vi "Decode DRV stand (SubVI).vi"(8 "error in (no error)":errorcluster, 9 "Excel Data":string[][](array[string]), 11 "SAP ID":string) -> (0 "error out":errorcluster, 1 "subarray":string[](array[string]), 3 "DRV stand":T1)   [LabVIEW 2018, in "Application.lvlib"]
uses:
  Application/Application.lvlib
  Application/DRV stand.ctl
panel:
  out "DriverID":string
  out "Name":string
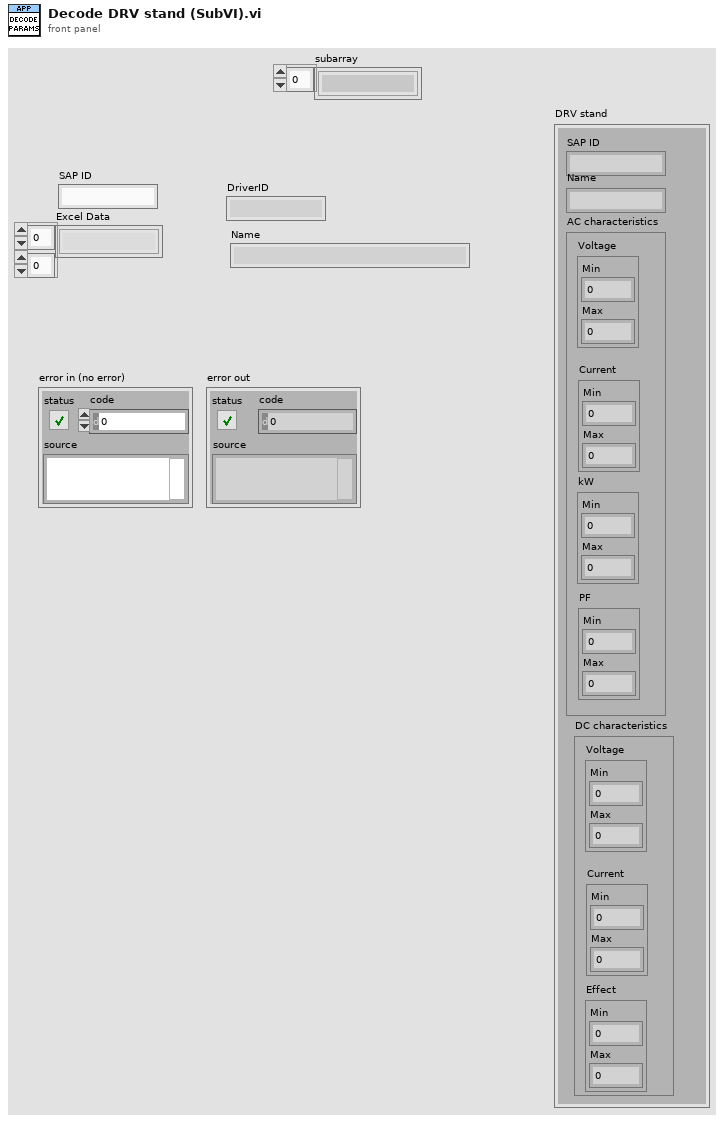
[diagram p1: front panel]
types:
  T1 = typedef "Application.lvlib/DRV stand.ctl" = cluster{"SAP ID":string, "Name":string, "AC characteristics":cluster{"Voltage":cluster{"Min":dbl, "Max":dbl}, "Current":cluster{"Min":dbl, "Max":dbl}, "kW":cluster{"Min":dbl, "Max":dbl}, "PF":cluster{"Min":dbl, "Max":dbl}}, "DC characteristics":cluster{"Voltage":cluster{"Min":dbl, "Max":dbl}, "Current":cluster{"Min":dbl, "Max":dbl}, "Effect":cluster{"Min":dbl, "Max":dbl}}}
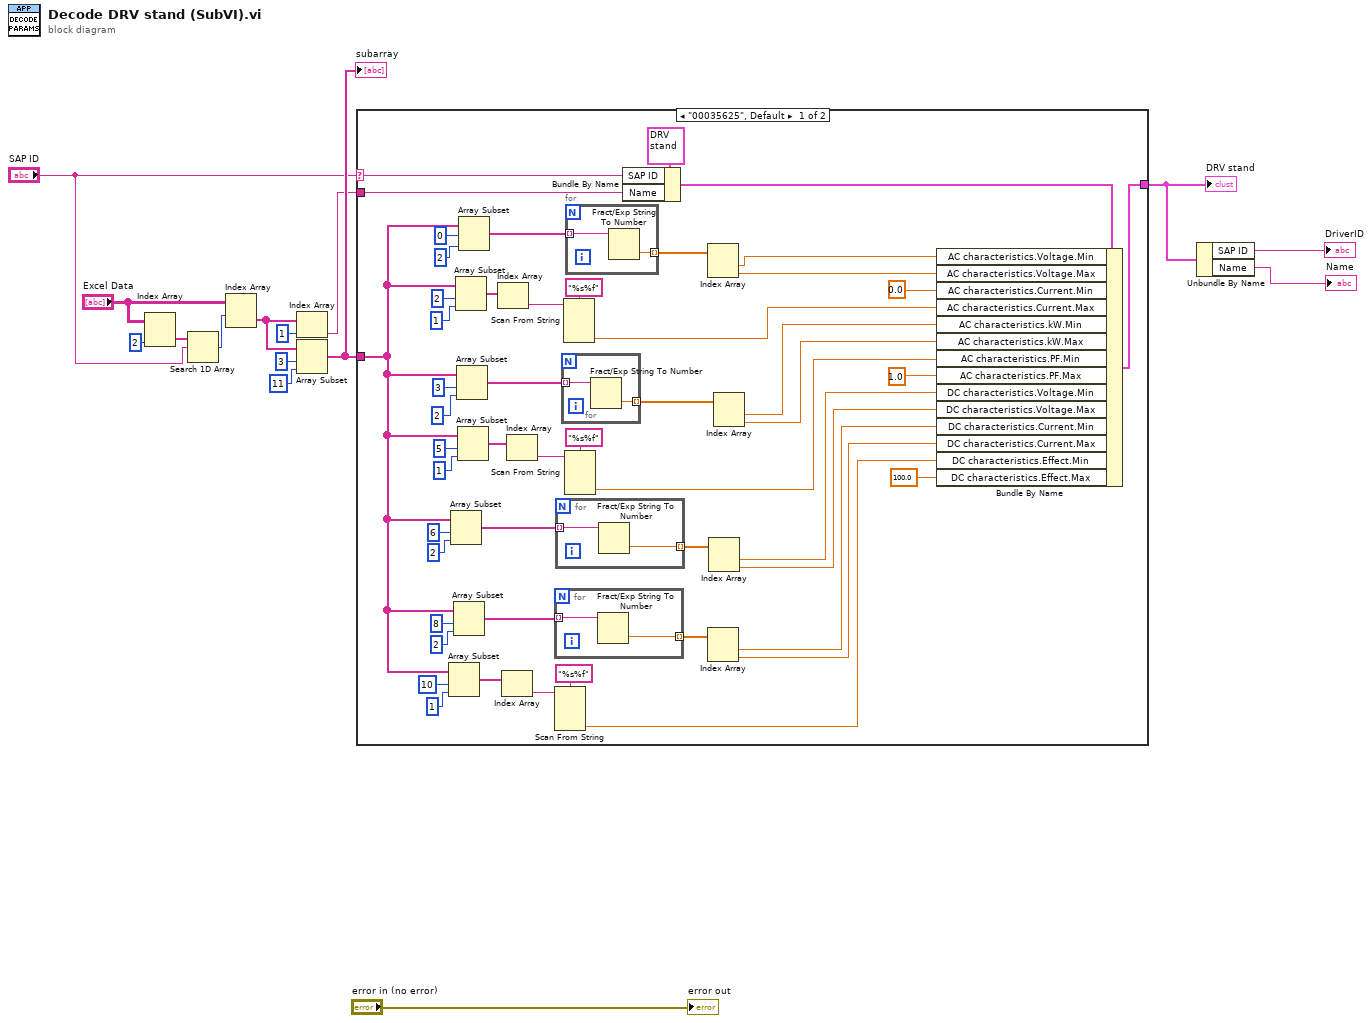
[diagram p0: block diagram]
diagram:
  n1 = Index Array(array="Excel Data", index (col)=2 ("disabled index (col)")) -> (element=w14:string[])  [unwired: 1 in]
  n2 = Search 1D Array(1D array=w14, element="SAP ID") -> (index of element=w13:i32)  [unwired: 1 in]
  n3 = Index Array(array="Excel Data", index (row)=w13) -> (element=w11:string[])  [unwired: 1 in]
  n4 = Index Array(array=w11, index=1) -> (element=w4:string)
  n5 = Array Subset(array=w11, index=3, length=11) -> (w7:string[])
  "subarray" <- w7
  n6 = case shown="\"00035625\", Default" "SAP ID" {
    selector: "SAP ID" -> [w18 _]
    tunnel: w7 -> [w19 _]
    tunnel: w4 -> [w17 _]
    tunnel: [w16 _] -> w1
    frame "00035625", Default {
      n7 = Array Subset(array=w19, index=10 ("length"), length=1) -> (w27:string[])
      n8 = Array Subset(array=w19, index=6 ("length"), length=2) -> (w40:string[])
      n9 = Array Subset(array=w19, index=8 ("length"), length=2) -> (w33:string[])
      n10 = Array Subset(array=w19, index=2 ("length"), length=1) -> (w57:string[])
      n11 = Array Subset(array=w19, index=3 ("length"), length=2) -> (w52:string[])
      n12 = Array Subset(array=w19, index=5 ("length"), length=1) -> (w45:string[])
      n13 = Array Subset(array=w19, index=0, length=2) -> (w65:string[])
      n14 = Index Array(array=w57) -> (element=w56:string)  [unwired: 1 in]
      n15 = Index Array(array=w27) -> (element=w26:string)  [unwired: 1 in]
      n16 = Index Array(array=w45) -> (element=w44:string)  [unwired: 1 in]
      n17 = for {
        tunnel: w33 -> [w68] mode=indexing
        tunnel: [w67] -> w34 mode=indexing
        n18 = Fract/Exp String To Number(string=w68) -> (number=w67:dbl)  [unwired: 3 in, 1 out]
      }
      n19 = Scan From String(format string="%s%f", input string=w26) -> (output 2=w24:dbl)  [unwired: 5 in, 3 out]
      n20 = for {
        tunnel: w40 -> [w70] mode=indexing
        tunnel: [w69] -> w39 mode=indexing
        n21 = Fract/Exp String To Number(string=w70) -> (number=w69:dbl)  [unwired: 3 in, 1 out]
      }
      n22 = for {
        tunnel: w52 -> [w72] mode=indexing
        tunnel: [w71] -> w51 mode=indexing
        n23 = Fract/Exp String To Number(string=w72) -> (number=w71:dbl)  [unwired: 3 in, 1 out]
      }
      n24 = Scan From String(format string="%s%f", input string=w56) -> (output 2=w55:dbl)  [unwired: 5 in, 3 out]
      n25 = Scan From String(format string="%s%f", input string=w44) -> (output 2=w43:dbl)  [unwired: 5 in, 3 out]
      n26 = for {
        tunnel: w65 -> [w74] mode=indexing
        tunnel: [w73] -> w64 mode=indexing
        n27 = Fract/Exp String To Number(string=w74) -> (number=w73:dbl)  [unwired: 3 in, 1 out]
      }
      n28 = Bundle By Name(cluster=T1 {"SAP ID"="", "Name"="", "AC characteristics"={"Voltage"={"Min"=0.0, "Max"=0.0}, "Current"={"Min"=0.0, "Max"=0.0}, "kW"={"Min"=0.0, "Max"=0.0}, "PF"={"Min"=0.0, "Max"=0.0}}, "DC characteristics"={"Voltage"={"Min"=0.0, "Max"=0.0}, "Current"={"Min"=0.0, "Max"=0.0}, "Effect"={"Min"=0.0, "Max"=0.0}}} ("DRV stand"), "SAP ID"=w18, "Name"=w17) -> (w25:T1)
      n29 = Index Array(array=w64) -> (element #1=w63:dbl, element #2=w62:dbl)  [unwired: 2 in]
      n30 = Index Array(array=w34) -> (element #1=w32:dbl, element #2=w31:dbl)  [unwired: 2 in]
      n31 = Index Array(array=w39) -> (element #1=w38:dbl, element #2=w37:dbl)  [unwired: 2 in]
      n32 = Index Array(array=w51) -> (element #1=w50:dbl, element #2=w49:dbl)  [unwired: 2 in]
      n33 = Bundle By Name(cluster=w25, "AC characteristics.Voltage.Min"=w63, "AC characteristics.Voltage.Max"=w62, "AC characteristics.Current.Min"=0.0, "AC characteristics.Current.Max"=w55, "AC characteristics.kW.Min"=w50, "AC characteristics.kW.Max"=w49, "AC characteristics.PF.Min"=w43, "AC characteristics.PF.Max"=1.0 ("AC characteristics.Current.Min"), "DC characteristics.Voltage.Min"=w38, "DC characteristics.Voltage.Max"=w37, "DC characteristics.Current.Min"=w32, "DC characteristics.Current.Max"=w31, "DC characteristics.Effect.Min"=w24, "DC characteristics.Effect.Max"=100.0) -> (w16:T1)
    }
    frame "false" {
    }
  }
  "DRV stand" <- w1
  n34 = Unbundle By Name(w1) -> ("SAP ID"=→"DriverID":string, "Name"=→"Name":string)
  "error out" <- "error in (no error)"
